vi "Example - Register endpoint.vi"() -> ()   [LabVIEW 2020, in "wamplv.lvlib"]
uses:
  wamplv.lvlib
  WAMP Client/WAMP Client.lvclass/WAMP Client.ctl
  86c89e9c-a710-438b-81a6-9e903d6b3f4b.vi
  c3cc1781-c523-44fe-81ce-48e472358bfc.vi
  WAMP Client/Private/SubVIs/Raise Internal Message.vi
  <vilib>/JDP Science/JSONtext/Variant to JSON Text.vi
  <vilib>/JDP Science/JSONtext/JSON text to Variant.vi
  <vilib>/Utility/error.llb/Error Cluster From Error Code.vi
  <vilib>/JDP Science/JSONtext/LVClass Serializer/JSONtext LVClass Serializer.lvclass
  WAMP Client/WAMP Client.lvclass
  Private/Invocation Request ID/Invocation Request ID.lvclass
panel:
  in  "Disconnect":bool caption="Publish Topic"
  out "ArgumentKw":string
  out "Arguments":string[](array[string])
  in  "Arguments to Return":string[](array[string])=["Hello", "World!"]
  in  "Endpoint name":string="test.endpoint"
  in  "Realm":string="default_realm"
  in  "Router Address":string="ws://localhost:8080/"
  # "Received Argumets"
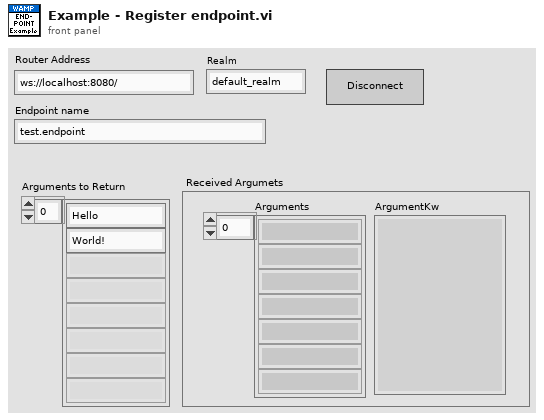
[diagram p1: front panel]
types:
  T1 = typedef "wamplv.lvlib/WAMP Client.lvclass/INVOCATION payload.ctl" = cluster{"Arguments":string, "ArgumentKw":string, "Procedure URI":string, "Details":string, "Registration ID":u64, "Invocation Request ID":refnum<class "Invocation Request ID.lvclass">}
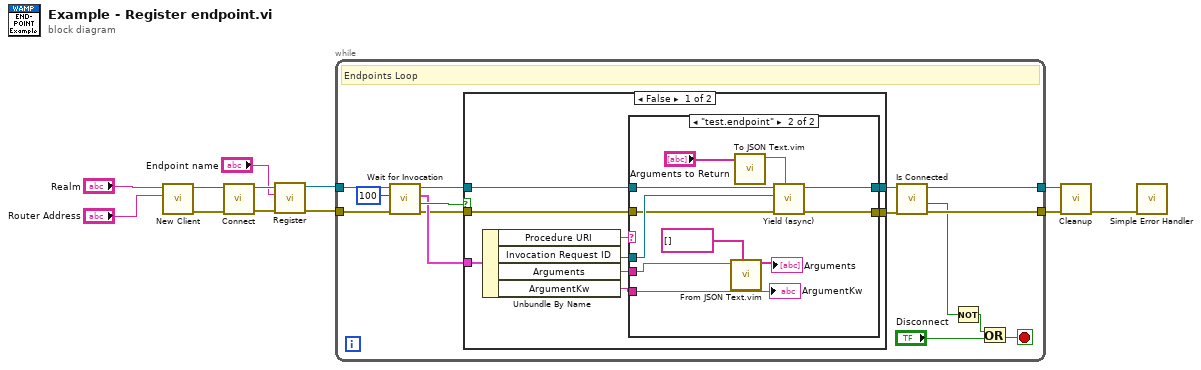
[diagram p0: block diagram]
diagram:
  n1 = call "New Client.vi"("Address"="Router Address", "Realm"="Realm") -> ("error out"=w8:errorcluster, "WAMP client out"=w10:refnum<class "WAMP Client.lvclass">)  [unwired: 8 in]
  n2 = call "Connect.vi"("error in"=w8, "WAMP Client in"=w10) -> ("error out"=w6:errorcluster, "WAMP Client out"=w5:refnum<class "WAMP Client.lvclass">)  [unwired: 8 in]
  n3 = call-dynamic "Register.vi"("Error in"=w6, "Procedure URI"="Endpoint name", "WAMP Client in"=w5) -> ("Error out"=w3:errorcluster, "WAMP Client out"=w2:refnum<class "WAMP Client.lvclass">)  [unwired: 6 in, 1 out]
  n4 = while {
    tunnel: w2 -> [w27]
    tunnel: w3 -> [w26]
    tunnel: [w18] -> w7
    tunnel: [w17] -> w1
    stop <- w14 stop-if-true
    # "Endpoints Loop"
    n5 = call "Wait for Invocation.vi"("error in (no error)"=w26, "timeout in ms (-1)"=100, "WAMP Client in"=w27) -> ("error out"=w21:errorcluster, "timed out?"=w24:bool, "WAMP Invocation"=w22:T1, "WAMP Client out"=w23:refnum<class "WAMP Client.lvclass">)  [unwired: 5 in]
    n6 = case shown="False" w24 {
      tunnel: w23 -> [w34 w51]
      tunnel: w22 -> [w36 _]
      tunnel: w21 -> [w32 w50]
      tunnel: [w31 w50] -> w19
      tunnel: [w30 w51] -> w20
      frame False {
        n7 = Unbundle By Name(w36) -> ("Procedure URI"=w35:string, "Invocation Request ID"=w33:refnum<class "Invocation Request ID.lvclass">, "Arguments"=w29:string, "ArgumentKw"=w28:string)
        n8 = case shown="\"test.endpoint\"" w35 {
          tunnel: w34 -> [w38 w49]
          tunnel: w33 -> [_ w48]
          tunnel: w32 -> [w37 w47]
          tunnel: [w37 w46] -> w31
          tunnel: [w38 w45] -> w30
          tunnel: w29 -> [_ w41]
          tunnel: w28 -> [_ w42]
          frame Default {
          }
          frame "test.endpoint" {
            n9 = call "From JSON Text.vim"("Data Type and Default Value"=string[] [] ("Arguments"), "JSON"=w41) -> ("Data out"=→"Arguments":string[])  [unwired: 8 in, 1 out]
            n10 = call "To JSON Text.vim"("Anything"="Arguments to Return") -> ("<JSON>"=w44:string)  [unwired: 9 in, 1 out]
            n11 = call "Yield (async).vi"("WAMP Client in"=w49, "wamplv.lvlib:Invocation Request.lvclass"=w48, "error in (no error)"=w47, "Arguments"=w44) -> ("WAMP Client out"=w45:refnum<class "WAMP Client.lvclass">, "error out"=w46:errorcluster)  [unwired: 5 in]
            "ArgumentKw" <- w42
          }
        }
      }
      frame True {
      }
    }
    n12 = call "Is Connected.vi"("error in"=w19, "WAMP Client in"=w20) -> ("error out"=w18:errorcluster, "Is Connected?"=w16:bool, "WAMP Client out"=w17:refnum<class "WAMP Client.lvclass">)  [unwired: 7 in]
    n13 = Not(x=w16) -> (.not. x?=w15:bool)
    n14 = Or(x=w15, y="Disconnect") -> (x .or. y?=w14:bool)
  }
  n15 = call-dynamic "Cleanup.vi"("error in"=w7, "WAMP Client in"=w1) -> ("error out"=w9:errorcluster)  [unwired: 8 in, 1 out]
  n16 = call <vilib>:"Simple Error Handler.vi"("error in (no error)"=w9) -> ()  [unwired: 4 in, 5 out]
